vi "ComdToConsole.vi"(7 "error in":errorcluster, 8 "command":string) -> (2 "error out":errorcluster, 3 "Disconnect?":bool)   [LabVIEW 2012]
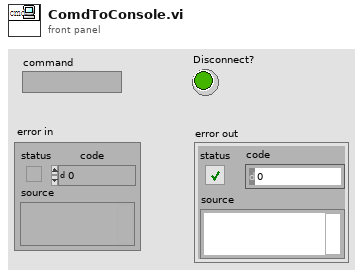
[diagram p1: front panel]
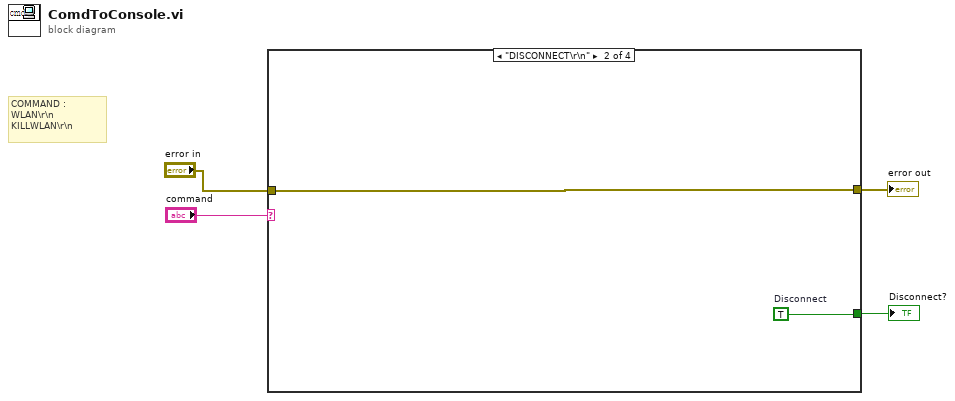
[diagram p0: block diagram]
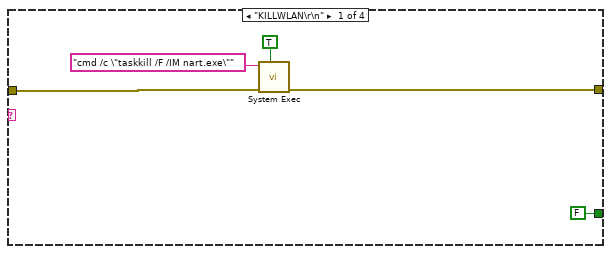
[diagram p2: hidden frame]
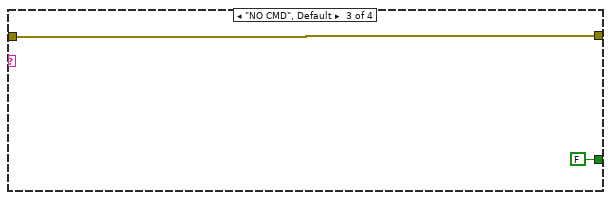
[diagram p3: hidden frame]
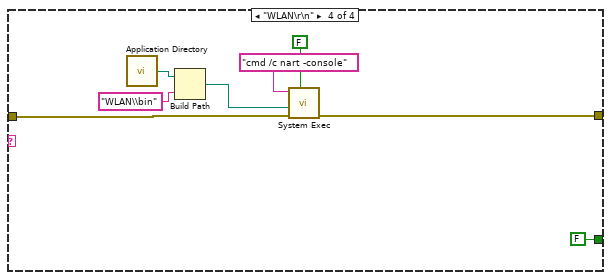
[diagram p4: hidden frame]
diagram:
  # "COMMAND :        \nWLAN\\r\\n\nKILLWLAN\\r\\n"
  n1 = case shown="\"DISCONNECT\\r\\n\"" "command" {
    tunnel: "error in" -> [w7 w11 w13 w19]
    tunnel: [w6 w11 w13 w18] -> w2
    tunnel: [FALSE ("Disconnect") w10 FALSE ("Disconnect") FALSE ("Disconnect")] -> w1
    frame "KILLWLAN\r\n" {
      n2 = call <vilib>:"System Exec.vi"("wait until completion? (T)"=TRUE, "error in (no error)"=w7, "command line"="cmd /c \"taskkill /F /IM nart.exe\"") -> ("error out"=w6:errorcluster)  [unwired: 5 in, 3 out]
    }
    frame "DISCONNECT\r\n" {
      w10 = TRUE  # Disconnect
    }
    frame "NO CMD", Default {
    }
    frame "WLAN\r\n" {
      n3 = call <vilib>:"Application Directory.vi"() -> ("Application Directory"=w21:path)
      n4 = Build Path(base path=w21, name or relative path="WLAN\\bin") -> (appended path=w17:path)
      n5 = call <vilib>:"System Exec.vi"("wait until completion? (T)"=FALSE, "error in (no error)"=w19, "working directory"=w17, "command line"="cmd /c nart -console") -> ("error out"=w18:errorcluster)  [unwired: 4 in, 3 out]
    }
  }
  "error out" <- w2
  "Disconnect?" <- w1
